vi "IPS120 WH0 - Send Command.vi"(3 "error in (no error)":errorcluster, 4 "Command String":string, 5 "VISA Address":refnum<visa-resource-name>) -> (0 "error out":errorcluster, 1 "Response String":string, 2 "VISA resource name out":refnum<visa-resource-name>)   [LabVIEW 2019]
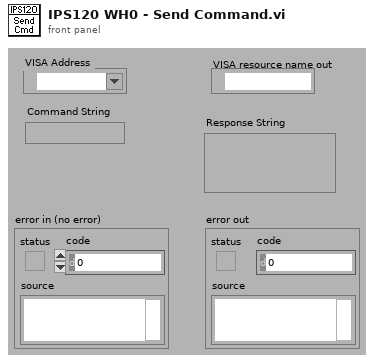
[diagram p1: front panel]
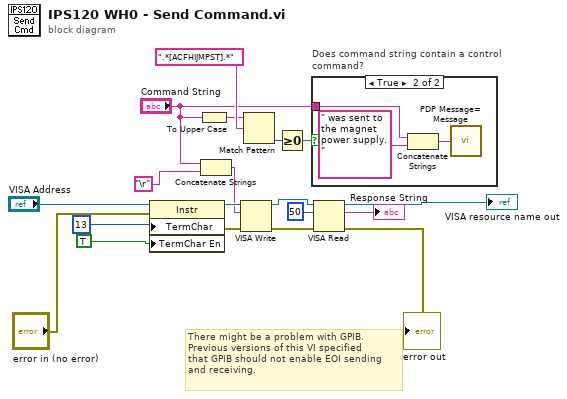
[diagram p0: block diagram]
diagram:
  # "There might be a problem with GPIB.\nPrevious versions of this VI specified\nthat GPIB should not enable EOI sending\nand receiving."
  n1 = property class="Instr"(reference="VISA Address", error in="error in (no error)", "TermChar"=u8 13 ("Message Based Settings:Termination Character"), "TermChar En"=TRUE ("Message Based Settings:Termination Character Enable")) -> (reference out=w11:refnum<visa-resource-name>, error out=w10:errorcluster)
  n2 = To Upper Case(1:"Command String") -> (0:w16:string)
  n3 = Concatenate Strings("Command String", "\r") -> (w2:string)
  n4 = VISA Write(VISA resource name=w11, write buffer=w2, error in (no error)=w10) -> (VISA resource name out=w13:refnum<visa-resource-name>, error out=w12:errorcluster)  [unwired: 1 out]
  n5 = Match Pattern(string=w16, regular expression=".*[ACFHIJMPST].*") -> (offset past match=w14:i32)  [unwired: 1 in, 3 out]
  n6 = Greater Or Equal To 0?(x=w14) -> (x >= 0?=w15:bool)
  n7 = case "Does command string contain a control command?" shown="True" w15 {
    tunnel: "Command String" -> [_ w22]
    frame False {
    }
    frame True {
      n8 = Concatenate Strings(w22, " was sent to the magnet power supply.") -> (w20:string)
      n9 = call "PDP Message= Message.vi"("Message"=w20) -> ()
    }
  }
  n10 = VISA Read(VISA resource name=w13, byte count=50, error in (no error)=w12) -> (VISA resource name out=→"VISA resource name out":refnum<visa-resource-name>, read buffer=→"Response String":string, error out=→"error out":errorcluster)  [unwired: 1 out]
